vi "연결ID (글로벌).vi"() -> ()   [LabVIEW 2014]
panel:
  in  "연결 ID":refnum<k5>
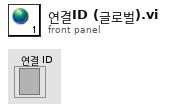
[diagram p1: front panel]
diagram:
